vi "First Description Paragraph.vi"(8 "Error In":errorcluster, 11 "Description":string) -> (0 "Error Out":errorcluster, 3 "First Paragraph":string)   [LabVIEW 2018, in "Scripts.lvlib"]
uses:
  Scripts.lvlib
  <vilib>/regexp/Match Regular Expression.xnode
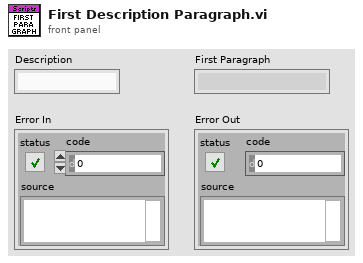
[diagram p1: front panel]
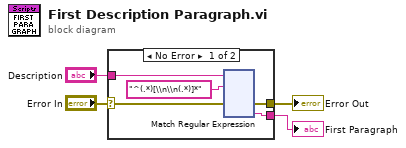
[diagram p0: block diagram]
diagram:
  n1 = case shown="No Error" "Error In" {
    selector: "Error In" -> [w5 w126]
    tunnel: "Description" -> [w9 _]
    tunnel: [w7 _] -> w3
    tunnel: [w6 w126] -> w2
    frame No Error {
      n2 = xnode "Match Regular Expression"("input string"=w9, "regular expression"="^(.*)[\\n\\n(.*)]*", "error in"=w5) -> ("error out"=w6:errorcluster, "submatch 1"=w7:string)  [unwired: 3 in, 4 out]
    }
    frame Error {
    }
  }
  "First Paragraph" <- w3
  "Error Out" <- w2
